vi "FestoCPX.getDiagnostics.vi"(1 "Festo error":u16) -> (0 "Festo error explanation":string)   [LabVIEW 2013]
panel:
  # "out"
  # "in"
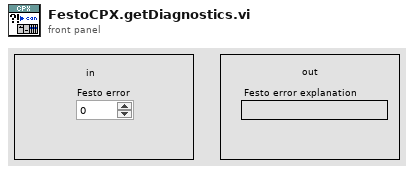
[diagram p1: front panel]
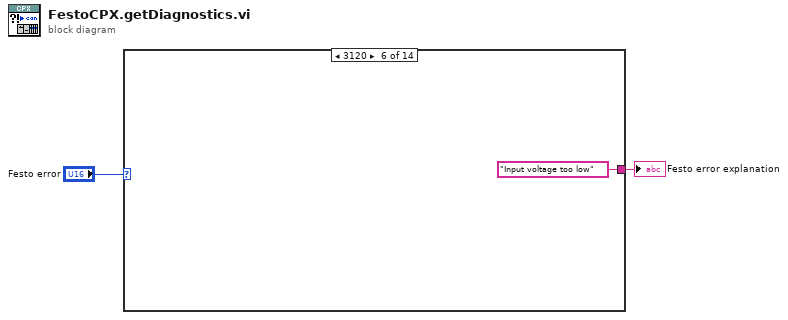
[diagram p0: block diagram]
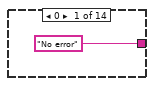
[diagram p2: hidden frame]
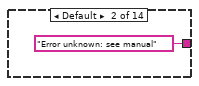
[diagram p3: hidden frame]
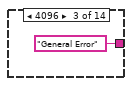
[diagram p4: hidden frame]
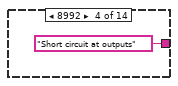
[diagram p5: hidden frame]
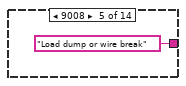
[diagram p6: hidden frame]
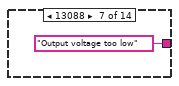
[diagram p7: hidden frame]
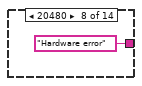
[diagram p8: hidden frame]
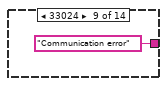
[diagram p9: hidden frame]
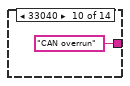
[diagram p10: hidden frame]
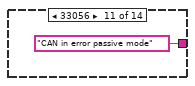
[diagram p11: hidden frame]
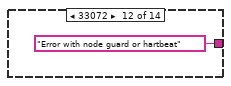
[diagram p12: hidden frame]
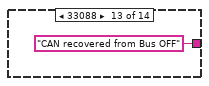
[diagram p13: hidden frame]
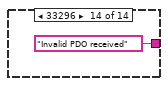
[diagram p14: hidden frame]
diagram:
  n1 = case shown="3120" "Festo error" {
    tunnel: ["No error" "Error unknown: see manual" "General Error" "Short circuit at outputs" "Load dump or wire break" "Input voltage too low" "Output voltage too low" "Hardware error" "Communication error" "CAN overrun" "CAN in error passive mode" "Error with node guard or hartbeat" "CAN recovered from Bus OFF" "Invalid PDO received"] -> w1
    frame 0 {
    }
    frame Default {
    }
    frame 4096 {
    }
    frame 8992 {
    }
    frame 9008 {
    }
    frame 12576 {
    }
    frame 13088 {
    }
    frame 20480 {
    }
    frame 33024 {
    }
    frame 33040 {
    }
    frame 33056 {
    }
    frame 33072 {
    }
    frame 33088 {
    }
    frame 33296 {
    }
  }
  "Festo error explanation" <- w1
